vi "Number of Obstructed Sectors.vi"(11 "Boolean Array":bool[](array[boolean])) -> (3 "Number of Obstructed Sectors":i32)   [LabVIEW 2009]
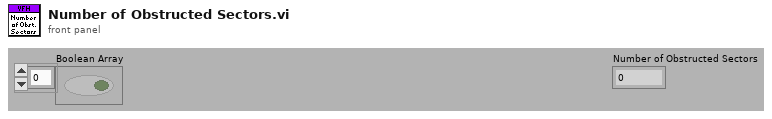
[diagram p1: front panel]
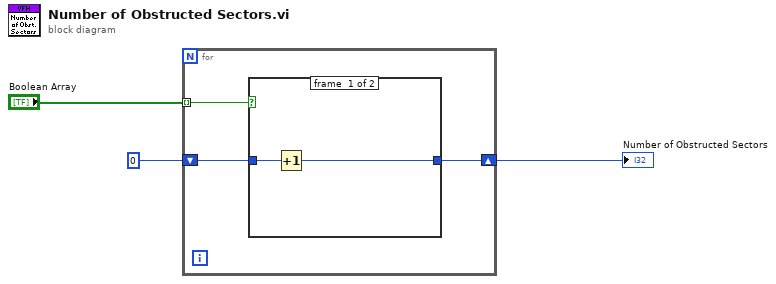
[diagram p0: block diagram]
diagram:
  n1 = for {
    tunnel: "Boolean Array" -> [w4] mode=indexing
    shift-right: [w5] -> w1
    shift-left: 0 -> [w6]
    n2 = case shown="True" w4 {
      tunnel: w6 -> [w8 w9]
      tunnel: [w7 w9] -> w5
      frame #0 {
        n3 = Increment(x=w8) -> (x+1=w7:i32)
      }
      frame #1 {
      }
    }
  }
  "Number of Obstructed Sectors" <- w1
